vi "Load HW from XML.vi"(8 "error in (no error)":errorcluster, 11 "Path":path) -> (0 "error out":errorcluster, 3 "All Hardware":refnum<class "Hardware Settings.lvclass">)   [LabVIEW 2017, in "Hardware Settings.lvclass"]
uses:
  Hardware Settings.lvclass
  <vilib>/Utility/xml.llb/Read From XML File(string).vi
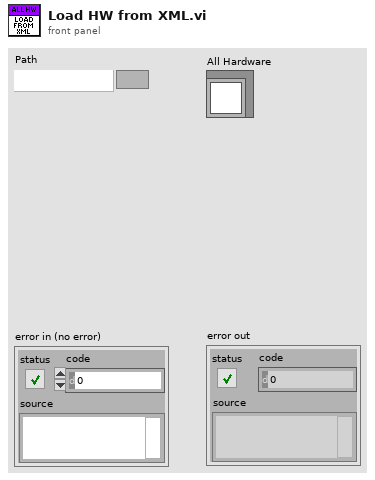
[diagram p1: front panel]
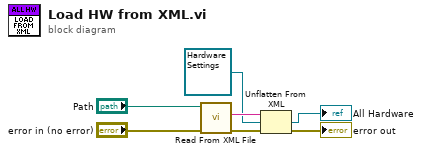
[diagram p0: block diagram]
diagram:
  n1 = call-poly <vilib>:"Read From XML File.vi"("error in (no error)"="error in (no error)", "XML File Path"="Path") -> ("error out"=w3:errorcluster, "XML Elements"=w5:string)  [unwired: 7 in, 1 out]
  n2 = Unflatten From XML(xml string=w5, type=refnum<class "Hardware Settings.lvclass"> refnum ("Hardware Settings.lvclass"), error in (no error)=w3) -> (value=→"All Hardware":refnum<class "Hardware Settings.lvclass">, error out=→"error out":errorcluster)
